vi "main.vi"() -> ()   [LabVIEW 2015]
uses:
  Telegram/Methods/TypeDefs/Message.ctl
panel:
  in  "Stop":bool
  out "ConnectionStatus":bool
  out "StatusLog":string
  out "Messages":T1[](array[typedef]) {"date" format="%<%I:%M:%S %p %x>T"}
  out "Error and Warning List":string
  # "myRIO+TelegramBOT Demo"
  # "update_id                from                               text                                         date                       chat_id                 type"
  # "Command list:\n\n/led#,Period(ms/us),DutyCycle(%) - Set LED 1-3 brightness, for example /led1,1000,50\n/led#, where # - number of LED (1-3). Returns User keyboard with on/off buttons\n/getweather,Ñity,Region - returns region weather data, for example /getweather,miami,us \n/gettime - returns current myRIO time"
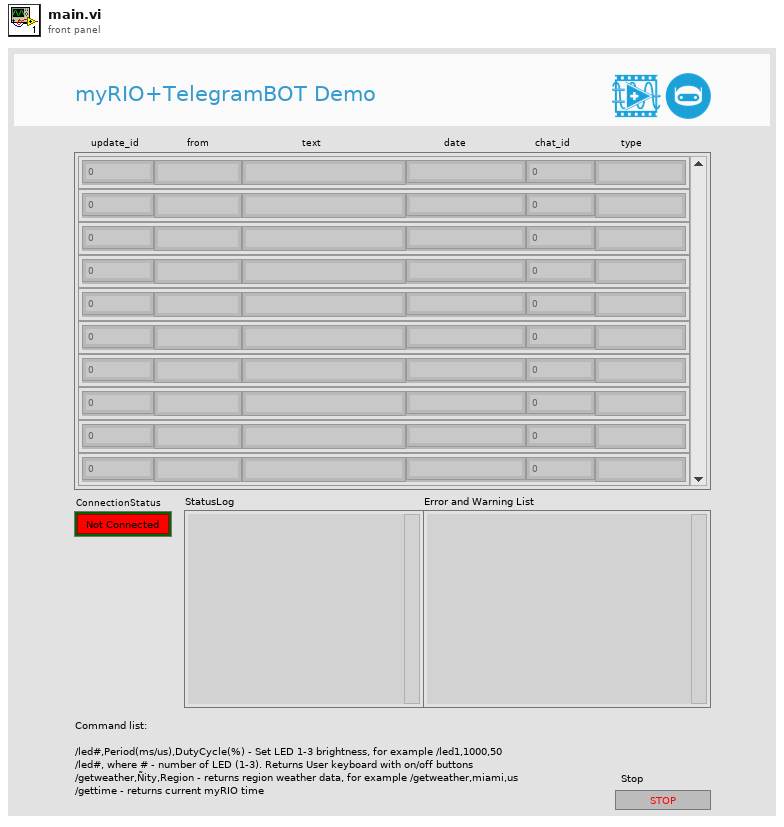
[diagram p1: front panel]
types:
  T1 = typedef "Message.ctl" = cluster{"update_id":u32, "from":string, "text":string, "date":timestamp, "chat_id":i32, "type":string, "reply_to_message.text":string, "message_id":u32}
  T2 = cluster{"Messages":refnum<queue>, "Errors":refnum<queue>}
  T3 = typedef "UpdateUniversal.ctl" = cluster{"update_id":u32, "message":cluster{"message_id":u32, "from":cluster{"id":u32, "first_name":string}, "chat":cluster{"id":i32, "first_name":string, "type":string}, "date":u32, "text":string, "reply_to_message":cluster{"message_id":u32, "from":cluster{"id":u32, "first_name":string}, "chat":cluster{"id":i32, "first_name":string, "type":string}, "date":u32, "text":string}}}[]
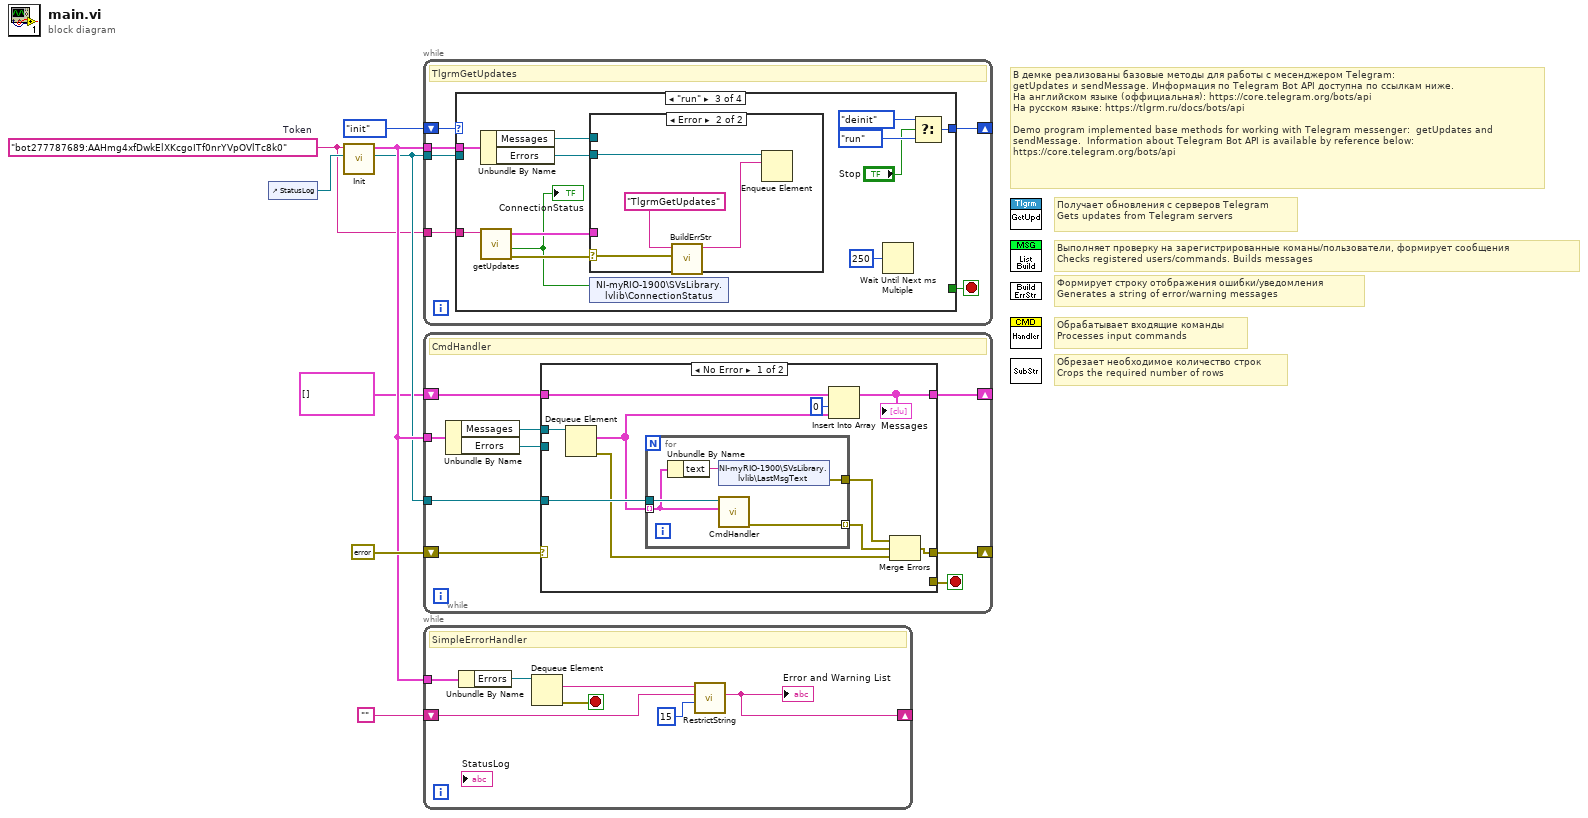
[diagram p0: block diagram]
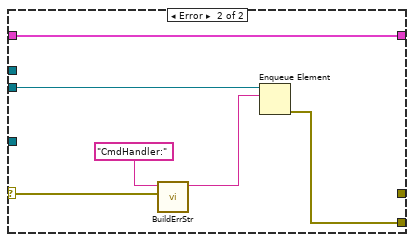
[diagram p2: hidden frame]
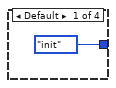
[diagram p3: hidden frame]
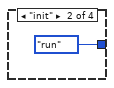
[diagram p4: hidden frame]
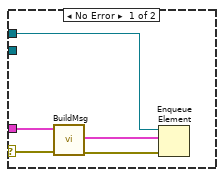
[diagram p5: hidden frame]
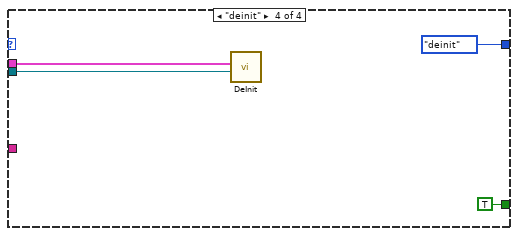
[diagram p6: hidden frame]
diagram:
  w1 = "bot277787689:AAHmg4xfDwkElXKcgoITf0nrYVpOVlTc8k0"  # Token
  # "В демке реализованы базовые методы для работы с месенджером Telegram:\ngetUpdates и sendMessage. Информация по Telegram Bot API доступна по ссылкам ниже.\nНа английском языке (оффициальная): https://core.telegram.org/bots/api\nНа русском языке: https://tlgrm.ru/docs/bots/api\n\nDemo program implemented base methods for working with Telegram messenger:  getUpdates and \nsendMessage.  Information about Telegram Bot API is available by reference below:\nhttps://core.telegram.org/bots/api"
  # "Обрезает необходимое количество строк\nCrops the required number of rows"
  # "Обрабатывает входящие команды\nProcesses input commands"
  # "Формирует строку отображения ошибки/уведомления\nGenerates a string of error/warning messages"
  # "Выполняет проверку на зарегистрированные команы/пользователи, формирует сообщения\nChecks registered users/commands. Builds messages"
  # "Получает обновления с серверов Telegram\nGets updates from Telegram servers"
  n1 = control-ref of="StatusLog"() -> (w5:refnum<vi>)
  n2 = call "Init.vi"("RefStringIn"=w5, "Token"=w1) -> ("GlobalDataRef"=w4:refnum<data-value>, "Queues"=w6:T2)  [unwired: 8 in]
  n3 = while {
    tunnel: w6 -> [w13]
    tunnel: w4 -> [w9]
    shift-right: [w12] -> _
    shift-left: enum16{"init", "run", "deinit"}."init" -> [w14]
    tunnel: w1 -> [w10]
    stop <- w11 stop-if-true
    # "TlgrmGetUpdates"
    n4 = case shown="\"run\"" w14 {
      tunnel: w13 -> [_ _ w25 w39]
      tunnel: w9 -> [_ _ _ w38]
      tunnel: [enum16{"init", "run", "deinit"}."init" enum16{"init", "run", "deinit"}."run" w26 enum16{"init", "run", "deinit"}."deinit"] -> w12
      tunnel: [_ _ _ TRUE ("Stop")] -> w11
      tunnel: w10 -> [_ _ w18 _]
      frame Default {
      }
      frame "init" {
      }
      frame "run" {
        n5 = Unbundle By Name(w25) -> ("Messages"=w22:refnum<queue>, "Errors"=w21:refnum<queue>)
        n6 = call "getUpdates.vi"("Token"=w18) -> ("error out"=w24:errorcluster, "ConnectionStatus"=w17:bool, "UpdateUniversal"=w23:T3)  [unwired: 7 in, 1 out]
        "ConnectionStatus" <- w17
        n7 = case shown="Error" w24 {
          selector: w24 -> [w31 w37]
          tunnel: w23 -> [w32 _]
          tunnel: w22 -> [w30 _]
          tunnel: w21 -> [_ w36]
          frame No Error {
            n8 = call "BuildMsg.vi"("ErrorIn"=w31, "Result"=w32) -> ("ErrorOut"=w33:errorcluster, "Messages"=w29:T1[])  [unwired: 8 in]
            n9 = Enqueue Element(queue=w30, element=w29, error in (no error)=w33) -> ()  [unwired: 1 in, 3 out]
          }
          frame Error {
            n10 = call "BuildErrStr.vi"("ErrorIn"=w37, "IinitString"="TlgrmGetUpdates") -> ("OutMsg"=w35:string)  [unwired: 9 in]
            n11 = Enqueue Element(queue=w36, element=w35) -> ()  [unwired: 2 in, 3 out]
          }
        }
        n12 = shared-variable "NI-myRIO-1900\\SVsLibrary.lvlib\\ConnectionStatus"(w17) -> ()  [unwired: 1 in, 1 out]
        n13 = Wait Until Next ms Multiple(millisecond multiple=u32 250) -> ()  [unwired: 1 out]
        n14 = Select(t=enum16{"init", "run", "deinit"}."deinit", s="Stop", f=enum16{"init", "run", "deinit"}."run") -> (s? t:f=w26:enum16{"init", "run", "deinit"})
      }
      frame "deinit" {
        n15 = call "DeInit.vi"("GlobalDataRef"=w38, "Queues"=w39) -> ()  [unwired: 10 in]
      }
    }
  }
  n16 = while {
    tunnel: w6 -> [w50]
    shift-right: [w46] -> _
    shift-left: errorcluster {"status"=FALSE, "code"=0, "source"=""} ("error IO") -> [w47]
    tunnel: w4 -> [w45]
    shift-right: [w43] -> _
    shift-left: T1[] [] -> [w42]
    stop <- w44 stop-if-true
    # "CmdHandler"
    n17 = Unbundle By Name(w50) -> ("Messages"=w49:refnum<queue>, "Errors"=w48:refnum<queue>)
    n18 = case shown="No Error" w47 {
      selector: w47 -> [_ w69]
      tunnel: w49 -> [w60 _]
      tunnel: w48 -> [_ w70]
      tunnel: [w57 _] -> w46
      tunnel: w45 -> [w59 _]
      tunnel: [_ w67] -> w44
      tunnel: [w56 w66] -> w43
      tunnel: w42 -> [w54 w66]
      frame No Error {
        n19 = Dequeue Element(queue=w60) -> (element=w55:T1[], error out=w52:errorcluster)  [unwired: 2 in, 2 out]
        n20 = for {
          tunnel: w55 -> [w63] mode=indexing
          tunnel: w59 -> [w65]
          tunnel: [w64] -> w58 mode=indexing
          tunnel: [w61] -> w51
          n21 = Unbundle By Name(w63) -> ("text"=w62:string)
          n22 = shared-variable "NI-myRIO-1900\\SVsLibrary.lvlib\\LastMsgText"(w62) -> (error out=w61:errorcluster)  [unwired: 1 in]
          n23 = call "CmdHandler.vi"("Message"=w63, "GlobalDataRef"=w65) -> ("Error"=w64:errorcluster)  [unwired: 9 in]
        }
        n24 = Insert Into Array(array=w54, index=0, new element=w55) -> (w56:T1[])
        "Messages" <- w56
        n25 = Merge Errors(w51, w58, w52) -> (w57:errorcluster)
      }
      frame Error {
        n26 = call "BuildErrStr.vi"("ErrorIn"=w69, "IinitString"="CmdHandler:") -> ("OutMsg"=w71:string)  [unwired: 9 in]
        n27 = Enqueue Element(queue=w70, element=w71) -> (error out=w67:errorcluster)  [unwired: 2 in, 2 out]
      }
    }
  }
  n28 = while {
    tunnel: w6 -> [w77]
    shift-right: [w73] -> _
    shift-left: "" -> [w74]
    stop <- w78 stop-if-true
    # "SimpleErrorHandler"
    n29 = Unbundle By Name(w77) -> ("Errors"=w76:refnum<queue>)
    n30 = Dequeue Element(queue=w76) -> (element=w75:string, error out=w78:errorcluster)  [unwired: 2 in, 2 out]
    n31 = call "RestrictString.vi"("NumberOfString"=15, "StringIn"=w74, "NewString"=w75) -> ("StringOut"=w73:string)  [unwired: 8 in]
    "Error and Warning List" <- w73
  }
